vi "Init Msg Attributes.vi"(6 "Msg Output":refnum<class "Msg Output.lvclass">, 9 "Msg Input":refnum<class "Msg Input.lvclass">, 10 "Msg":refnum<class "Msg.lvclass">) -> (0 "Error out":errorcluster, 2 "Msg Attributes":refnum<data-value>)   [LabVIEW 2020, in "jettl.lvlib"]
uses:
  jettl.lvlib
  Relation.ctl
  Teller.ctl
  Msg Output/Msg Output.lvclass
  Msg Input/Msg Input.lvclass
  Msg/Msg.lvclass
  Msg Attributes.ctl
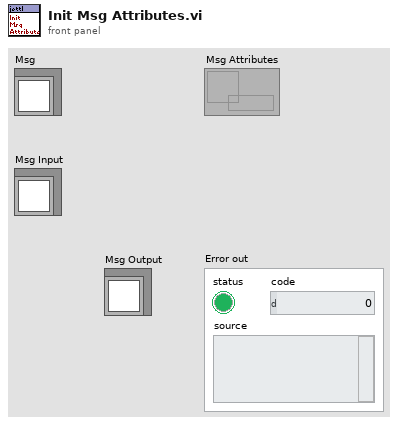
[diagram p1: front panel]
types:
  T1 = typedef "jettl.lvlib/Msg Attributes.ctl" = cluster{"Msg":refnum<class "Msg.lvclass">, "Msg Input":refnum<class "Msg Input.lvclass">, "Msg Output":refnum<class "Msg Output.lvclass">, "Teller":T2}
  T2 = typedef "jettl.lvlib/Teller.ctl" = cluster{"Absolute Time":timestamp, "Relative Time":dbl, "Alias":string, "Relation":T3}
  T3 = typedef "jettl.lvlib/Relation.ctl" = enum16{"Self", "Parent", "Child"}
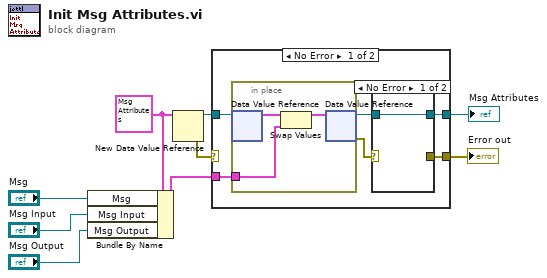
[diagram p0: block diagram]
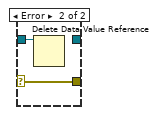
[diagram p2: hidden frame]
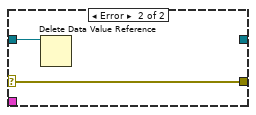
[diagram p3: hidden frame]
diagram:
  w4 = T1 {"Msg"=refnum, "Msg Input"=refnum, "Msg Output"=refnum, "Teller"={"Absolute Time"=timestamp(0 s since 1904-01-01), "Relative Time"=0.0, "Alias"="", "Relation"=enum."Self"}} ("Msg Attributes")
  n1 = Bundle By Name(cluster=w4, "Msg"="Msg", "Msg Input"="Msg Input", "Msg Output"="Msg Output") -> (w5:T1)
  n2 = New Data Value Reference(data value=w4) -> (data value reference=w9:refnum<data-value>, error out=w7:errorcluster)  [unwired: 1 in]
  n3 = case shown="No Error" w7 {
    selector: w7 -> [_ w22]
    tunnel: w9 -> [w15 w23]
    tunnel: [w14 _] -> w8
    tunnel: [w11 w22] -> w6
    tunnel: w5 -> [w10 _]
    frame No Error {
      n4 = in-place {
        in-place-border: w10 -> [w16]
        n5 = in-place-dvr #1(w15) -> (w18:T1)  [unwired: 1 out]
        n6 = Swap Values(12:w18, 14:w16) -> (1:w17:T1)  [unwired: 1 in, 1 out]
        n7 = in-place-dvr #1(w17) -> (w13:refnum<data-value>, w12:errorcluster)
      }
      n8 = case shown="No Error" w12 {
        selector: w12 -> [_ w21]
        tunnel: [w19 _] -> w14
        tunnel: w13 -> [w19 w20]
        tunnel: [_ w21] -> w11
        frame No Error {
        }
        frame Error {
          n9 = Delete Data Value Reference(data value reference=w20) -> ()  [unwired: 1 in, 2 out]
        }
      }
    }
    frame Error {
      n10 = Delete Data Value Reference(data value reference=w23) -> ()  [unwired: 1 in, 2 out]
    }
  }
  "Msg Attributes" <- w8
  "Error out" <- w6
